vi "Adder2.vi"() -> (8 "Adder2":refnum<class "Adder2.lvclass">)   [LabVIEW 2017, in "Adder2.lvclass"]
uses:
  Adder2.lvclass
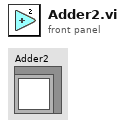
[diagram p1: front panel]
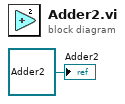
[diagram p0: block diagram]
diagram:
  "Adder2" <- refnum<class "Adder2.lvclass"> refnum ("Adder2.lvclass")
